vi "Main Launcher.vi"() -> ()   [LabVIEW 2010, in "Launcher.lvlib"]
uses:
  Launcher.lvlib
  Module/Template Module.lvlib
  Error Handler/Error Handler.lvlib
  UI 1/UI 1.lvlib
panel:
  out "error out":errorcluster
  in  "error in (no error)":errorcluster
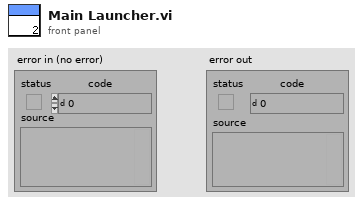
[diagram p1: front panel]
types:
  T1 = typedef "Launcher.lvlib/Event Message Cluster.ctl" = cluster{"Module Event":refnum<user-event>, "Error Event":refnum<user-event>, "Shutdown Event":refnum<user-event>}
  T2 = typedef "Template Module.lvlib/User Event Message Enum.ctl" = enum16{"Event 1"}
  T3 = typedef "Error Handler.lvlib/User Event Message Enum.ctl" = enum16{"Event 1"}
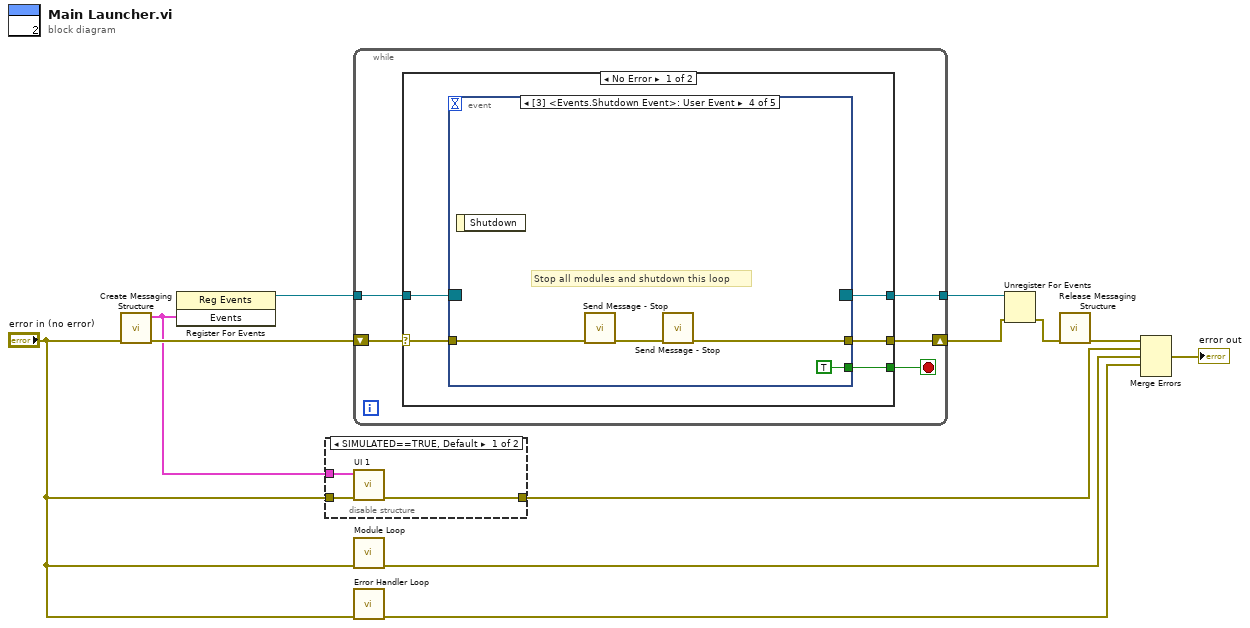
[diagram p0: block diagram]
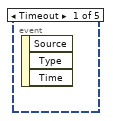
[diagram p3: hidden frame]
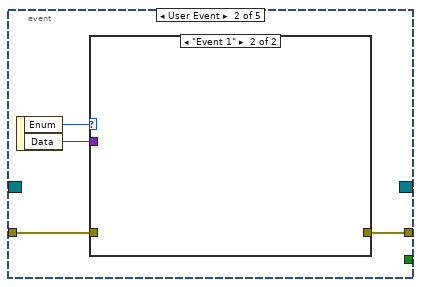
[diagram p4: hidden frame]
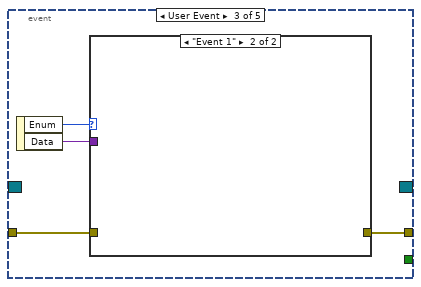
[diagram p6: hidden frame]
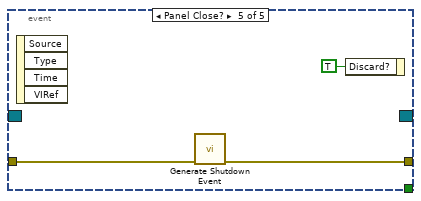
[diagram p8: hidden frame]
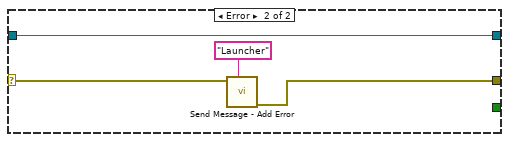
[diagram p9: hidden frame]
diagram:
  n1 = call "Create Messaging Structure.vi"("error in (no error)"="error in (no error)") -> ("error out"=w12:errorcluster, "Events"=w5:T1)  [unwired: 9 in]
  n2 = register-events(w5) -> (reference out=w11:refnum<event-registration>)  [unwired: 2 in, 1 out]
  n3 = disable-structure shown="SIMULATED==TRUE, Default" {
    disable-tunnel: "error in (no error)" -> [w15 _]
    disable-tunnel: w5 -> [w14 _]
    disable-tunnel: [w13 _] -> w3
    frame condition #0 (active) {
      n4 = call "UI 1.vi"("error in (no error)"=w15, "Event Refs"=w14) -> ("error out"=w13:errorcluster)  [unwired: 9 in]
    }
    frame condition #1 {
      # "Place modules for real hardware here"
    }
  }
  n5 = while {
    shift-right: [w17] -> w9
    shift-left: w12 -> [w20]
    tunnel: w11 -> [w19]
    tunnel: [w18] -> w10
    stop <- w16 stop-if-true
    n6 = case shown="No Error" w20 {
      selector: w20 -> [w23 w46]
      tunnel: w19 -> [w25 w44]
      tunnel: [w24 w44] -> w18
      tunnel: [w22 w45] -> w17
      tunnel: [w21 _] -> w16
      frame No Error {
        n7 = event shown="[3] <Events.Shutdown Event>: User Event" {
          selector: w25 -> [_ _ _ _ _]
          dyn-events: [_ _ _ _ _] -> w24
          timeout: _ -> [_ _ _ _ _]
          tunnel: w23 -> [_ w28 w33 w38 w41]
          tunnel: [_ w27 w32 w36 w40] -> w22
          tunnel: [_ _ _ TRUE _] -> w21
          event Timeout {
            n8 = event-data() -> ()  [unwired: 1 in, 3 out]
          }
          event User Event {
            n9 = event-data() -> ("Enum"=w29:T2, "Data"=w26:variant)  [unwired: 1 in]
            n10 = case shown="\"Event 1\"" w29 {
              tunnel: w28 -> [w30 _]
              tunnel: [w30 _] -> w27
              tunnel: w26 -> [_ _]
              frame Default {
              }
              frame "Event 1" {
              }
            }
          }
          event User Event {
            n11 = event-data() -> ("Enum"=w34:T3, "Data"=w31:variant)  [unwired: 1 in]
            n12 = case shown="\"Event 1\"" w34 {
              tunnel: w33 -> [w35 _]
              tunnel: [w35 _] -> w32
              tunnel: w31 -> [_ _]
              frame Default {
              }
              frame "Event 1" {
              }
            }
          }
          event User Event {
            # "Stop all modules and shutdown this loop"
            n13 = event-data() -> ()  [unwired: 1 in, 1 out]
            n14 = call "Send Message - Stop.vi"("error in (no error)"=w38) -> ("error out"=w37:errorcluster)  [unwired: 10 in]
            n15 = call "Send Message - Stop.vi"("error in (no error)"=w37) -> ("error out"=w36:errorcluster)  [unwired: 10 in]
          }
          event Panel Close? {
            n16 = event-data() -> ()  [unwired: 1 in, 4 out]
            n17 = call "Generate Shutdown Event.vi"("error in (no error)"=w41) -> ("error out"=w40:errorcluster)  [unwired: 10 in]
            n18 = event-data("Discard?"=TRUE) -> ()  [unwired: 1 in, 1 out]
          }
        }
      }
      frame Error {
        n19 = call "Send Message - Add Error.vi"("Source"="Launcher", "Error to Handle"=w46) -> ("error out"=w45:errorcluster)  [unwired: 9 in]
      }
    }
  }
  n20 = call "Module Loop.vi"("error in (no error)"="error in (no error)") -> ("error out"=w2:errorcluster)  [unwired: 10 in]
  n21 = call "Error Handler Loop.vi"("error in (no error)"="error in (no error)") -> ("error out"=w1:errorcluster)  [unwired: 10 in]
  n22 = Unregister For Events(event registration refnum=w10, error in=w9) -> (error out=w8:errorcluster)
  n23 = call "Release Messaging Structure.vi"("error in (no error)"=w8) -> ("error out"=w7:errorcluster)  [unwired: 10 in]
  n24 = Merge Errors(w7, w3, w2, w1) -> (→"error out":errorcluster)  [unwired: 1 in]
